vi "Update Motor Config Control Settings.vi"(5 "2#电机配置数据":T1 {"电流（A）" format="%.1f"}, 7 "1#电机配置数据":T1 {"电流（A）" format="%.1f"}, 8 "error in (no error)":errorcluster, 10 "电机2配置ref":refnum<vi>, 11 "电机1配置ref":refnum<vi>) -> (0 "error out":errorcluster)   [LabVIEW 2018]
uses:
  Ctls/MotorConfig.ctl
  Ctls/MotroConfigData.ctl
  Ctls/MagType.ctl
panel:
  in  "电机2配置":T2
  in  "电机1配置":T2
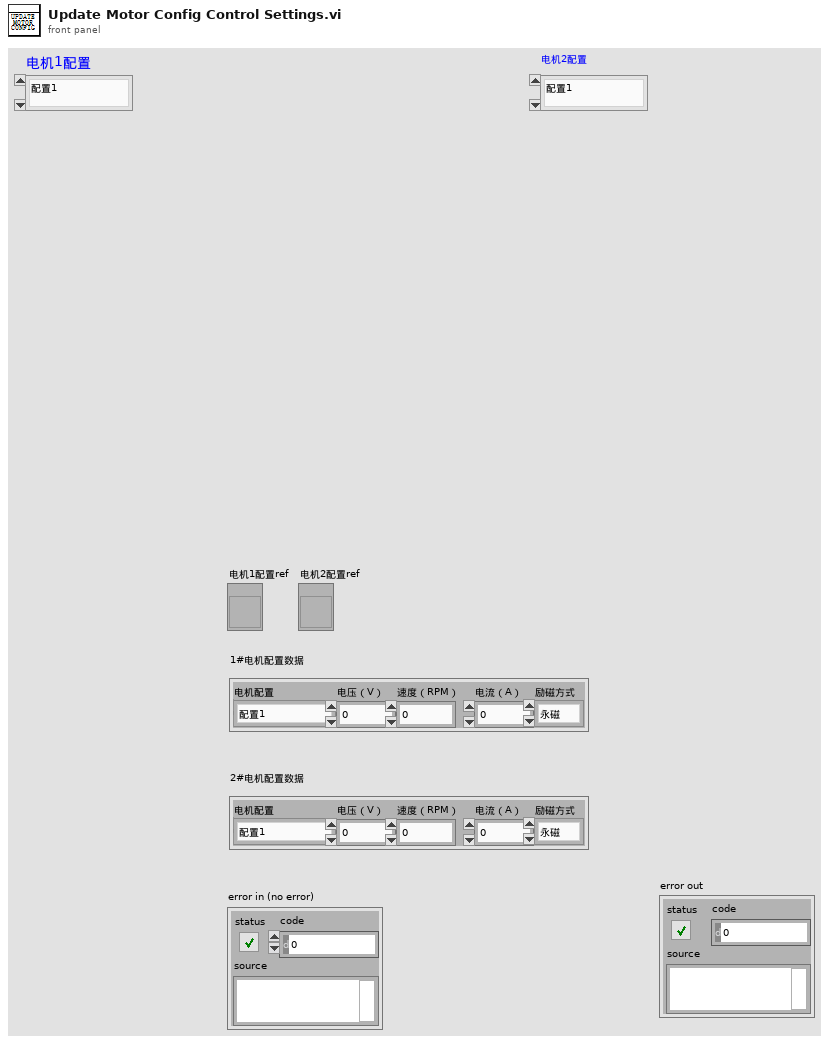
[diagram p1: front panel]
types:
  T1 = typedef "MotroConfigData.ctl" = cluster{"电机配置":T2, "电压（V）":u16, "速度（RPM）":u16, "电流（A）":u16, "励磁方式":T3}
  T2 = typedef "MotorConfig.ctl" = enum16{"配置1", "配置2", "配置3", "配置4"}
  T3 = typedef "MagType.ctl" = enum16{"永磁", "励磁"}
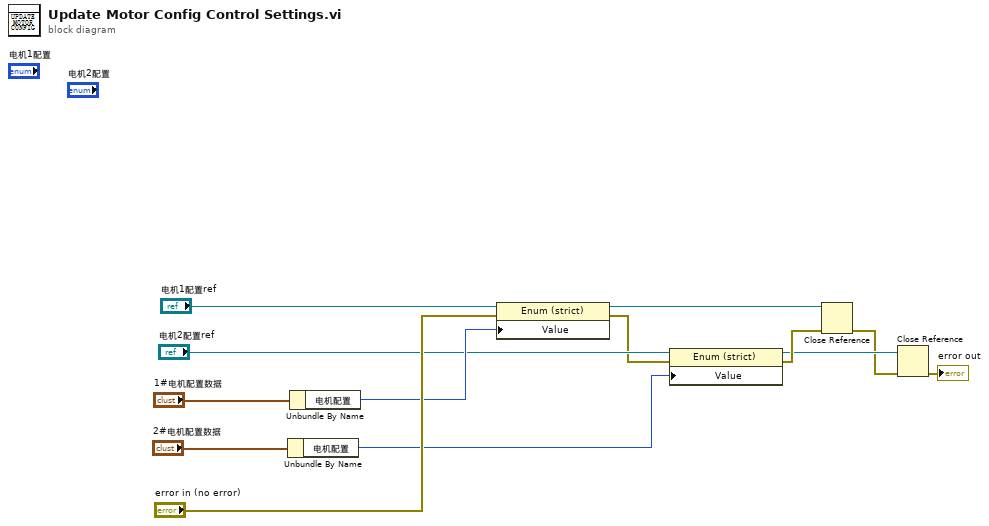
[diagram p0: block diagram]
diagram:
  n1 = Unbundle By Name("2#电机配置数据") -> ("电机配置"=w6:T2)
  n2 = Unbundle By Name("1#电机配置数据") -> ("电机配置"=w9:T2)
  n3 = property class="Enum (strict)"(reference="电机1配置ref", error in="error in (no error)", "Value"=w9) -> (reference out=w4:refnum<vi>, error out=w7:errorcluster)
  n4 = property class="Enum (strict)"(reference="电机2配置ref", error in=w7, "Value"=w6) -> (reference out=w3:refnum<vi>, error out=w5:errorcluster)
  n5 = Close Reference(reference=w4, error in (no error)=w5) -> (error out=w2:errorcluster)
  n6 = Close Reference(reference=w3, error in (no error)=w2) -> (error out=→"error out":errorcluster)
